vi "source_ramp_voltage.vi"(0 "Input parameters":T1={"Measurement type"=enum."Debug", "Sensor type"=enum."HPK_8in_271ch", "Identifier"="test.txt", "Open after execution?"=FALSE, "Plot after execution?"=FALSE, "Display channel"=0, "Voltage Delay (s)"=0.5, "Switch Delay (s)"=0.01, "VISA resource name source"="", "VISA resource name DMM"="", "VISA resource name LCR"="", "Compliance  Level (A)"=10.0, "Voltage Limit (V)"=1000.0, "Data storage location"="", "Scan voltages"="", "Use source as DMM?"=FALSE, "LCR signal frequenzy (Hz)"=10.0, "DMM device"=enum."Keithley2001", "Sampling number"=1, "Use env. sensors on"=enum."Sensirion sht1x/7x", "Switchboard Handle"=0, "Use Switchboard"=FALSE, "LCR signal voltage (V)"=10000.0, "Repeat"=1, "Scan voltages IV"="", "Scan voltages CV"="", "Hex pad numbers?"=FALSE, "Set measurement type"=enum."Debug", "Custom pad scan"="", "IV voltage Delay (s)"=0.5, "CV voltage Delay (s)"=0.5, "Needle measurement?"=FALSE, "Comments"="test.txt", "LCR signal frequenzy (kHz)"=10.0, "Compliance  Level (uA)"=10.0, "Open Correction Array"=array2304x3[6912 elements], "Current set voltage"=0.0, "Last set voltage"=0.0, "Current channel"=0, "Last OpenCorrection index"=-1, "Total curr/vltg every x steps"=10, "Current channel iteration"=0, "No CV corrections"=FALSE, "Mapfile"="", "Corrfile"="", "IV voltage file"=path "", "CV voltage file"=path "", "IV Switch Delay (s)"=0.01, "CV Switch Delay (s)"=0.01, "Invert polarity"=FALSE, "Set debug dirs"=FALSE, "Is n on p"=FALSE, "Source interlock?"=TRUE, "Voltage file used?"=FALSE, "Pad mask"="", "Mask pad above (uA)"=1.0, "LCR device"=enum."LCR_E4980", "Source device"=enum."Source_2410", "HexPlot binary path"="", "PadReductionFactor"=1.0, "Temperature degC"="", "Fluence [neq]"="", "Annealing [min]"=""} {"CV Switch Delay (s)" format="%#_13g"; "IV Switch Delay (s)" format="%#_13g"; "Last set voltage" format="%#_13g"; "Current set voltage" format="%#_13g"; "CV voltage Delay (s)" format="%#_13g"; "IV voltage Delay (s)" format="%#_13g"; "Voltage Limit (V)" format="%#_13g"; "Voltage Delay (s)" format="%#_13g"; "Switch Delay (s)" format="%#_13g"}, 7 "Target voltage (V)":dbl, 9 "Compliance Current (A)":dbl=0.1, 11 "error in (no error)":errorcluster, 12 "Current source voltage reference":refnum<vi>, 13 "Stop":refnum<vi>) -> (4 "VISA resource name out":refnum<visa-resource-name>, 6 "Current voltage out (V)":dbl, 8 "Aborted?":bool, 15 "error out":errorcluster)   [LabVIEW 2020]
doc: "Ramps voltage up or down in specified step size."
uses:
  input_params.ctl
  <instrlib>/Keithley 648X Series/Keithley 648X Series.lvlib
  <instrlib>/Keithley 24XX/Keithley 24XX.lvlib
panel:
  out "Actual voltage":dbl
  out "Tot. current":dbl
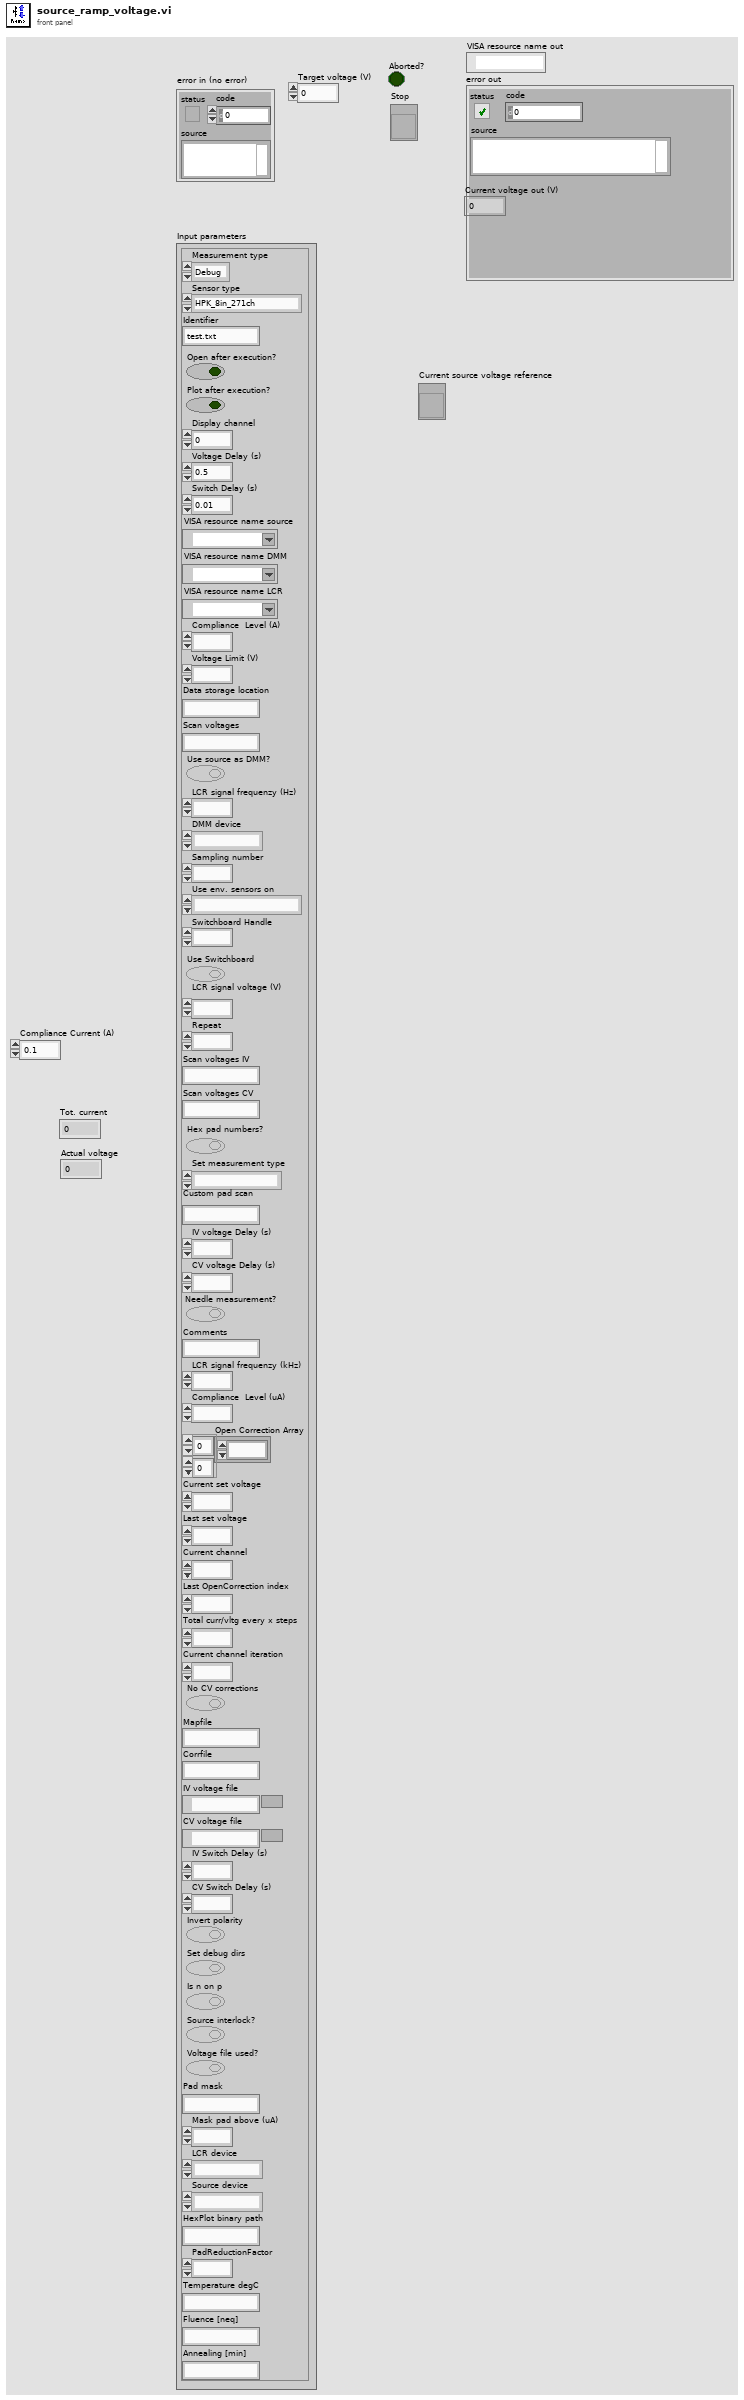
[diagram p1: front panel]
types:
  T1 = typedef "input_params.ctl" = cluster{"Measurement type":enum16{"IV", "CV", "Debug", "Test_contact"}, "Sensor type":enum16{"HPK_6in_135ch", "HPK_8in_271ch", "IFX_8in_256ch", "Diode", "HPK_6in_239ch", "Full_Matrix", "HPK_8in_271ch_full", "LumiCal", "HPK_8in_444ch", "HPK_8in_198ch_2019", "HPK_8in_MGW_LD_full", "HPK_8in_MGW_LD_a_type_top", "HPK_8in_MGW_LD_a_type_bottom", "HPK_8in_MGW_LD_b_type_left", "HPK_8in_MGW_LD_b_type_right", "HPK_8in_MGW_LD_c_type_left", "HPK_8in_MGW_LD_c_type_right", "HPK_8in_MGW_HD_full", "HPK_8in_MGW_HD_a_type_top", "HPK_8in_MGW_HD_a_type_bottom", "HPK_8in_MGW_HD_b_type_left", "HPK_8in_MGW_HD_b_type_right", "HPK_8in_MGW_HD_c_type_left", "HPK_8in_MGW_HD_c_type_right", "CALICE_6in_256ch"}, "Identifier":string, "Open after execution?":bool, "Plot after execution?":bool, "Display channel":i32, "Voltage Delay (s)":dbl, "Switch Delay (s)":dbl, "VISA resource name source":refnum<visa-resource-name>, "VISA resource name DMM":refnum<visa-resource-name>, "VISA resource name LCR":refnum<visa-resource-name>, "Compliance  Level (A)":dbl, "Voltage Limit (V)":dbl, "Data storage location":string, "Scan voltages":string, "Use source as DMM?":bool, "LCR signal frequenzy (Hz)":dbl, "DMM device":enum16{"Keithley2001", "Keithley2450", "Keithley2410", "Keithley6485", "Keithley6487", "Keithley6517"}, "Sampling number":i32, "Use env. sensors on":enum16{"Sensirion sht1x/7x", "Switch Matrix", "Probecard"}, "Switchboard Handle":u32, "Use Switchboard":bool, "LCR signal voltage (V)":dbl, "Repeat":i32, "Scan voltages IV":string, "Scan voltages CV":string, "Hex pad numbers?":bool, "Set measurement type":enum16{"IV", "CV", "Debug", "Test_contact", "IV+CV"}, "Custom pad scan":string, "IV voltage Delay (s)":dbl, "CV voltage Delay (s)":dbl, "Needle measurement?":bool, "Comments":string, "LCR signal frequenzy (kHz)":dbl, "Compliance  Level (uA)":dbl, "Open Correction Array":dbl[][], "Current set voltage":dbl, "Last set voltage":dbl, "Current channel":i32, "Last OpenCorrection index":i32, "Total curr/vltg every x steps":i32, "Current channel iteration":i32, "No CV corrections":bool, "Mapfile":string, "Corrfile":string, "IV voltage file":path, "CV voltage file":path, "IV Switch Delay (s)":dbl, "CV Switch Delay (s)":dbl, "Invert polarity":bool, "Set debug dirs":bool, "Is n on p":bool, "Source interlock?":bool, "Voltage file used?":bool, "Pad mask":string, "Mask pad above (uA)":dbl, "LCR device":enum16{"LCR_E4980", "AGILENT_4263X"}, "Source device":enum16{"Source_2410", "Source_6487", "Source_2470"}, "HexPlot binary path":string, "PadReductionFactor":dbl, "Temperature degC":string, "Fluence [neq]":string, "Annealing [min]":string}
  T2 = enum16{"Source_2410", "Source_6487", "Source_2470"}
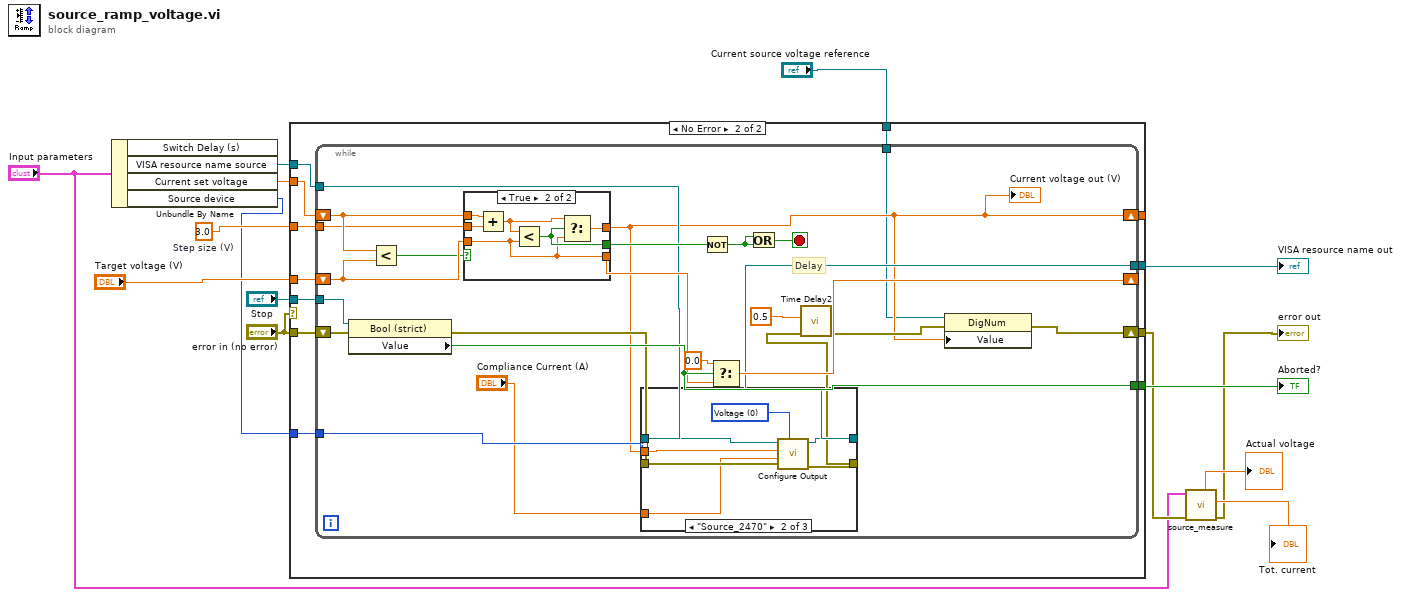
[diagram p0: block diagram]
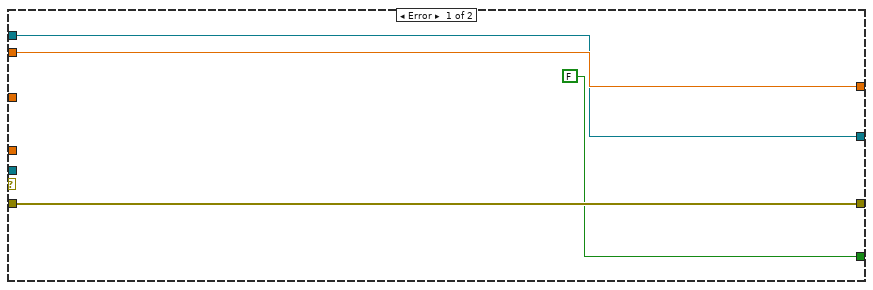
[diagram p2: hidden frame]
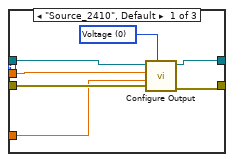
[diagram p3: hidden frame]
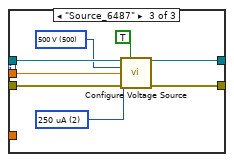
[diagram p4: hidden frame]
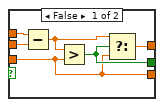
[diagram p5: hidden frame]
diagram:
  w8 = 3.0  # Step size (V)
  n1 = Unbundle By Name("Input parameters") -> ("VISA resource name source"=w10:refnum<visa-resource-name>, "Current set voltage"=w9:dbl, "Source device"=w7:T2)  [unwired: 1 out]
  n2 = case shown="No Error" "error in (no error)" {
    tunnel: "error in (no error)" -> [w18 w31]
    tunnel: "Target voltage (V)" -> [_ w24]
    tunnel: w9 -> [w19 w25]
    tunnel: w10 -> [w17 w30]
    tunnel: [w17 w29] -> w14
    tunnel: [w18 w28] -> w4
    tunnel: [w19 w23] -> _
    tunnel: "Stop" -> [_ w27]
    tunnel: [FALSE ("Value") w26] -> w11
    tunnel: w8 -> [_ w22]
    tunnel: w7 -> [_ w21]
    tunnel: "Current source voltage reference" -> [_ w20]
    frame Error {
    }
    frame No Error {
      n3 = while {
        shift-right: [w35] -> w28
        shift-left: w31 -> [w43]
        shift-right: [w33] -> w23
        shift-left: w25 -> [w50]
        tunnel: w30 -> [w42]
        tunnel: [w41] -> w29
        tunnel: w27 -> [w51]
        shift-right: [w44] -> _
        shift-left: w24 -> [w49]
        tunnel: [w47] -> w26
        tunnel: w22 -> [w39]
        tunnel: w21 -> [w38]
        tunnel: w20 -> [w32]
        stop <- w54 stop-if-true
        # "Delay"
        n4 = property class="Bool (strict)"(reference=w51, error in=w43) -> (error out=w40:errorcluster, "Value"=w47:bool)  [unwired: 1 out]
        n5 = Less?(x=w50, y=w49) -> (x < y?=w48:bool)
        n6 = case shown="True" w48 {
          tunnel: w49 -> [w78 w84]
          tunnel: w39 -> [w82 w88]
          tunnel: w50 -> [w83 w89]
          tunnel: [w80 w86] -> w33
          tunnel: [w79 w85] -> w53
          tunnel: [w78 w84] -> w45
          frame False {
            n7 = Subtract(x=w83, y=w82) -> (x-y=w81:dbl)
            n8 = Greater?(x=w81, y=w78) -> (0:w79:bool)
            n9 = Select(t=w81, s=w79, f=w78) -> (s? t:f=w80:dbl)
          }
          frame True {
            n10 = Add(x=w89, y=w88) -> (x+y=w87:dbl)
            n11 = Less?(x=w87, y=w84) -> (x < y?=w85:bool)
            n12 = Select(t=w87, s=w85, f=w84) -> (s? t:f=w86:dbl)
          }
        }
        "Current voltage out (V)" <- w33
        n13 = case shown="\"Source_2470\"" w38 {
          tunnel: w42 -> [w62 w69 w77]
          tunnel: [w58 w65 w76] -> w41
          tunnel: w33 -> [w61 w68 w75]
          tunnel: w40 -> [w60 w67 w74]
          tunnel: [w59 w66 w73] -> w36
          tunnel: "Compliance Current (A)" -> [w56 w63 _]
          frame "Source_2410", Default {
            w57 = u16 0 items=["Voltage", "Current"] ("Source Mode  (0: Voltage)")
            n14 = call <instrlib>:"Configure Output.vi"("Source Mode  (0: Voltage)"=w57, "error in (no error)"=w60, "Compliance  Level (0.1)"=w56, "Output Level (0)"=w61, "VISA resource name"=w62) -> ("error out"=w59:errorcluster, "VISA resource name out"=w58:refnum<visa-resource-name>)  [unwired: 5 in]
          }
          frame "Source_2470" {
            w64 = u16 0 items=["Voltage", "Current"] ("Source Mode  (0: Voltage)")
            n15 = call <instrlib>:"Configure Output.vi"("Source Mode  (0: Voltage)"=w64, "error in (no error)"=w67, "Compliance  Level (0.1)"=w63, "Output Level (0)"=w68, "VISA resource name"=w69) -> ("error out"=w66:errorcluster, "VISA resource name out"=w65:refnum<visa-resource-name>)  [unwired: 5 in]
          }
          frame "Source_6487" {
            w70 = u16 2 items=["25 mA", "2.5 mA", "250 uA", "25 uA"] ("Current Limit (25 mA)")
            w71 = u16 500 items=["10 V"=10, "50 V"=50, "500 V"=500] ("Voltage Source Range (10 V)")
            n16 = call <instrlib>:"Configure Voltage Source.vi"("VISA resource name"=w77, "Enable Voltage Source (F: Disable)"=TRUE, "Voltage Source Range (10 V)"=w71, "Voltage Level (0 V)"=w75, "Current Limit (25 mA)"=w70, "error in (no error)"=w74) -> ("VISA resource name out"=w76:refnum<visa-resource-name>, "error out"=w73:errorcluster)  [unwired: 8 in]
          }
        }
        n17 = Not(x=w53) -> (.not. x?=w52:bool)
        n18 = Select(t=0.0 ("Target voltage (V)"), s=w47, f=w45) -> (s? t:f=w44:dbl)
        n19 = Or(x=w52, y=w52) -> (x .or. y?=w54:bool)
        n20 = call "Time Delay2"("error in (no error)"=w36, "Delay Time (s)"=0.5 ("Delay (s)")) -> ("error out"=w34:errorcluster)  [unwired: 9 in]
        n21 = property class="DigNum"(reference=w32, error in=w34, "Value"=w33) -> (error out=w35:errorcluster)  [unwired: 1 out]
      }
    }
  }
  "VISA resource name out" <- w14
  "Aborted?" <- w11
  n22 = call "source_measure.vi"("error in (no error)"=w4, "Input parameters"="Input parameters") -> ("error out"=→"error out":errorcluster, "Total current"=→"Tot. current":dbl, "Actual voltage"=→"Actual voltage":dbl)  [unwired: 5 in, 2 out]
